vi "GraphArrayCreate.vi"(0 "Current A":dbl(knob) caption="Current A [mA]" min=0.0 max=50.0 step=0.01 scale=0.0..50.0 scale format="%#.3f", 1 "Power Source":refnum<visa-resource-name>, 2 "Commutator":refnum<visa-resource-name>, 3 "Multimeter":refnum<visa-resource-name>, 5 "Voltage  B":dbl(knob) caption="Voltage B [V]" min=0.0 max=50.0 step=0.01 scale=0.0..50.0 scale format="%#.3f", 7 "Max. transistor power":dbl=5.0 caption="Max. transistor power [mW]" min=5.0 max=150.0 step=5.0, 9 "Number of meas. points":i32) -> (8 "XY Graph":cluster{"Voltage Array":dbl[], "Ic Array":dbl[]}(graph), 15 "Cluster":cluster{dbl[], dbl[]})   [LabVIEW 2021]
panel:
  out "Ic Array":dbl[](array[numeric])
  out "Uc Array":dbl[](array[numeric])
  out "HP34401":dbl format="%#.3e"
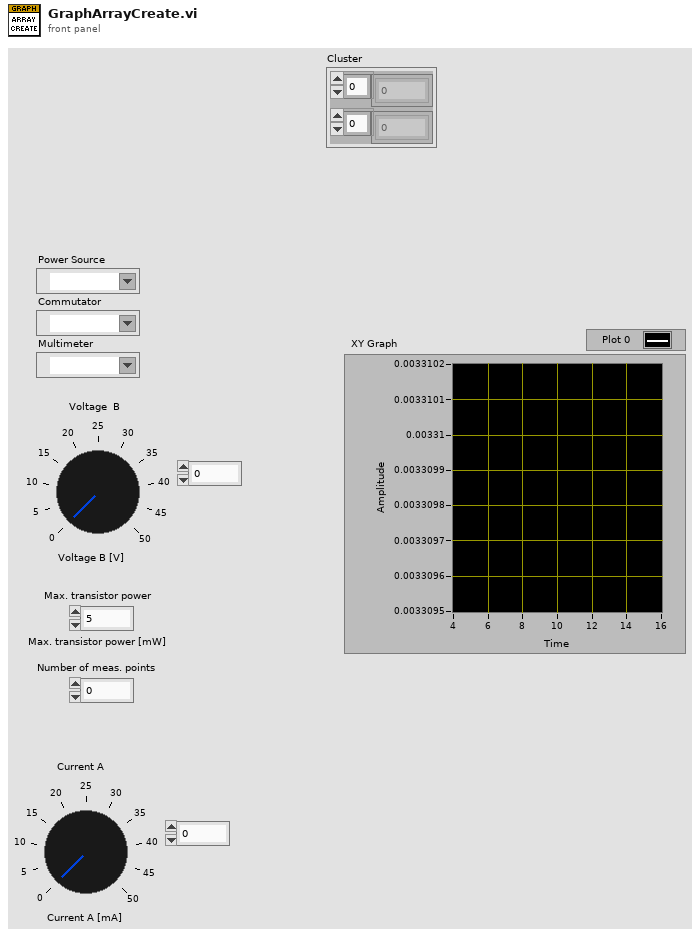
[diagram p1: front panel]
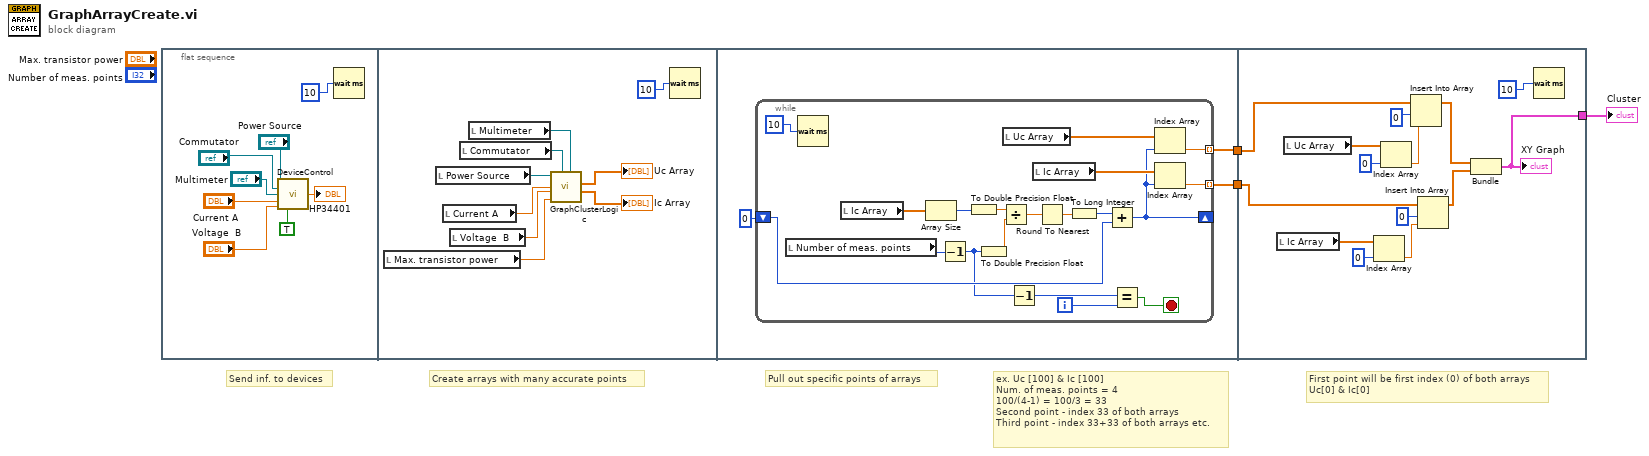
[diagram p0: block diagram]
diagram:
  # "Pull out specific points of arrays"
  # "Send inf. to devices"
  # "Create arrays with many accurate points"
  # "First point will be first index (0) of both arrays\nUc[0] & Ic[0]"
  # "ex. Uc [100] & Ic [100]\nNum. of meas. points = 4\n100/(4-1) = 100/3 = 33\nSecond point - index 33 of both arrays\nThird point - index 33+33 of both arrays etc."
  n1 = flat-sequence {
    tunnel: [w22] -> w3
    tunnel: [w21] -> w2
    tunnel: w3 -> [w56]
    tunnel: w2 -> [w52]
    tunnel: [w44] -> w1
    frame #0 {
      n2 = call "DeviceControl.vi"("Power Source"="Power Source", "Commutator"="Commutator", "Multimeter"="Multimeter", "Current A"="Current A", "Voltage  B"="Voltage  B", "PSU A or B"=TRUE) -> ("HP34401"=→"HP34401":dbl)  [unwired: 9 in]
      n3 = Wait (ms)(milliseconds to wait=u32 10) -> ()  [unwired: 1 out]
    }
    frame #1 {
      n4 = local read "Max. transistor power"() -> (w15:dbl)
      n5 = local read "Power Source"() -> (w20:refnum<visa-resource-name>)
      n6 = local read "Current A"() -> (w13:dbl)
      n7 = local read "Voltage  B"() -> (w14:dbl)
      n8 = local read "Commutator"() -> (w19:refnum<visa-resource-name>)
      n9 = local read "Multimeter"() -> (w18:refnum<visa-resource-name>)
      n10 = call "GraphClusterLogic.vi"("Multimeter"=w18, "Commutator"=w19, "Max. transistor power"=w15, "Voltage  B"=w14, "Current A"=w13, "Power Source"=w20) -> ("Ic Array"=→"Ic Array":dbl[], "Uc Array"=→"Uc Array":dbl[])  [unwired: 4 in]
      n11 = Wait (ms)(milliseconds to wait=u32 10) -> ()  [unwired: 1 out]
    }
    frame #2 {
      n12 = while {
        shift-right: [w24] -> _
        shift-left: 0 -> [w36]
        tunnel: [w31] -> w21 mode=indexing
        tunnel: [w28] -> w22 mode=indexing
        i -> [w35]
        stop <- w34 stop-if-true
        n13 = local read "Number of meas. points"() -> (w37:i32)
        n14 = Wait (ms)(milliseconds to wait=u32 10) -> ()  [unwired: 1 out]
        n15 = local read "Ic Array"() -> (w42:dbl[])
        n16 = Array Size(array=w42) -> (size(s)=w38:i32)
        n17 = Decrement(x=w37) -> (x-1=w26:i32)
        n18 = To Double Precision Float(number=w38) -> (double precision float=w39:dbl)
        n19 = To Double Precision Float(number=w26) -> (double precision float=w40:dbl)
        n20 = Divide(x=w39, y=w40) -> (x/y=w41:dbl)
        n21 = local read "Uc Array"() -> (w30:dbl[])
        n22 = Decrement(x=w26) -> (x-1=w25:i32)
        n23 = local read "Ic Array"() -> (w32:dbl[])
        n24 = Round To Nearest(number=w41) -> (nearest integer value=w33:dbl)
        n25 = To Long Integer(number=w33) -> (32bit integer=w29:i32)
        n26 = Add(x=w29, y=w36) -> (x+y=w24:i32)
        n27 = Equal?(x=w25, y=w35) -> (x = y?=w34:bool)
        n28 = Index Array(array=w30, index=w24) -> (element=w28:dbl)
        n29 = Index Array(array=w32, index=w24) -> (element=w31:dbl)
      }
    }
    frame #3 {
      n30 = local read "Ic Array"() -> (w49:dbl[])
      n31 = local read "Uc Array"() -> (w46:dbl[])
      n32 = Index Array(array=w49, index=0) -> (element=w48:dbl)
      n33 = Index Array(array=w46, index=0) -> (element=w45:dbl)
      n34 = Insert Into Array(array=w56, index=0, new element=w45) -> (w54:dbl[])
      n35 = Insert Into Array(array=w52, index=0, new element=w48) -> (w53:dbl[])
      n36 = Bundle(w54, w53) -> (w44:cluster{dbl[], dbl[]})  [unwired: 1 in]
      "XY Graph" <- w44
      n37 = Wait (ms)(milliseconds to wait=u32 10) -> ()  [unwired: 1 out]
    }
  }
  "Cluster" <- w1
